vi "strip cursor fragment regex tests.vi"() -> ()   [LabVIEW 2018]
uses:
  <vilib>/regexp/Match Regular Expression.xnode
panel:
  out "whole match 4":string
  out "whole match 3":string
  out "whole match 2":string
  out "whole match":string
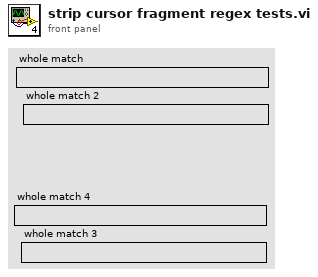
[diagram p1: front panel]
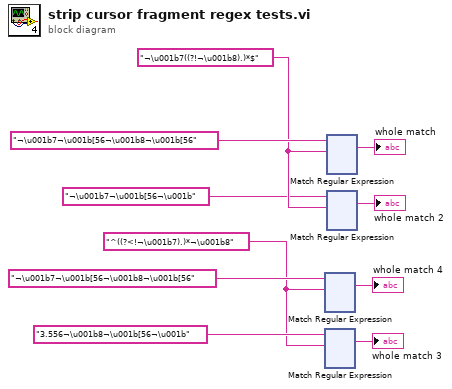
[diagram p0: block diagram]
diagram:
  w1 = "^((?<!¬\u001b7).)*¬\u001b8" ("search string")
  w7 = "¬\u001b7((?!¬\u001b8).)*$" ("search string")
  n1 = xnode "Match Regular Expression"("input string"="¬\u001b7¬\u001b[56¬\u001b8¬\u001b[56" ("search string"), "regular expression"=w1) -> ("whole match"=→"whole match 4":string)  [unwired: 4 in, 4 out]
  n2 = xnode "Match Regular Expression"("input string"="3.556¬\u001b8¬\u001b[56¬\u001b" ("search string"), "regular expression"=w1) -> ("whole match"=→"whole match 3":string)  [unwired: 4 in, 4 out]
  n3 = xnode "Match Regular Expression"("input string"="¬\u001b7¬\u001b[56¬\u001b8¬\u001b[56" ("search string"), "regular expression"=w7) -> ("whole match"=→"whole match":string)  [unwired: 4 in, 4 out]
  n4 = xnode "Match Regular Expression"("input string"="¬\u001b7¬\u001b[56¬\u001b" ("search string"), "regular expression"=w7) -> ("whole match"=→"whole match 2":string)  [unwired: 4 in, 4 out]
